vi "f(a).vi"(11 "x":u16) -> (3 "数值":u16)   [LabVIEW 2016, in "数据传输系统.lvlib"]
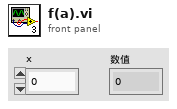
[diagram p1: front panel]
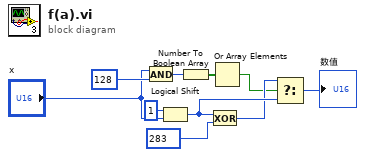
[diagram p0: block diagram]
diagram:
  n1 = And(x="x", y=u16 128 ("0x80 2")) -> (x .and. y?=w1:u16)
  n2 = Logical Shift(y=i8 1, x="x") -> (x << y=w6:u16)
  n3 = Number To Boolean Array(number=w1) -> (Boolean array=w2:bool[])
  n4 = Exclusive Or(1:u16 283 ("0x011b 2"), 2:w6) -> (0:w5:u16)
  n5 = Or Array Elements(Boolean array=w2) -> (logical OR=w3:bool)
  n6 = Select(t=w5, s=w3, f=w6) -> (s? t:f=→"数值":u16)
